vi "Format Fiducial Data.vi"(8 "error in":errorcluster, 9 "Module-Chuck Fiducials":T5(array[cluster]), 10 "Worktable":refnum<class "WorkTable Class.lvclass">, 11 "Console Log in":refnum<class "Console Log.lvclass">) -> (0 "error out":errorcluster, 2 "Formatted Fiducial Data":string, 3 "Console Log out":refnum<class "Console Log.lvclass">)   [LabVIEW 2011, in "Console Log.lvclass"]
uses:
  Console Log.lvclass
  Shared Components/Utils/Type Definitions/Fiducial Image.ctl
  Shared Components/Vec3d Class/Vec3d Class.lvclass
  Shared Components/Utils/Type Definitions/Physical Image.ctl
  <vilib>/vision/Image Controls.llb/IMAQ Image.ctl
  Shared Components/Utils/Type Definitions/Fiducial with Source.ctl
  Shared Components/WorkTable Class/WorkTable Class.lvclass
  Shared Components/Config Manager Class/Type Definitions/Part Type.ctl
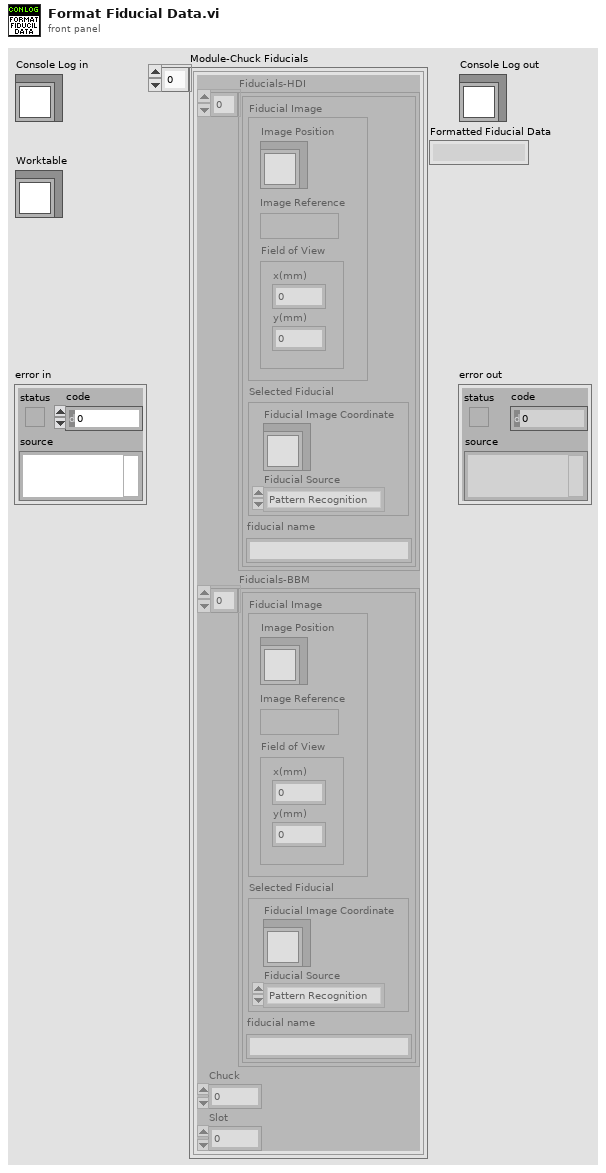
[diagram p1: front panel]
types:
  T1 = typedef "Fiducial Image.ctl" = cluster{"Fiducial Image":T2, "Selected Fiducial":T4, "fiducial name":string}
  T2 = typedef "Physical Image.ctl" = cluster{"Image Position":refnum<class "Vec3d Class.lvclass">, "Image Reference":T3, "Field of View":cluster{"x(mm)":dbl, "y(mm)":dbl}}
  T3 = typedef "IMAQ Image.ctl" = refnum<image>
  T4 = typedef "Fiducial with Source.ctl" = cluster{"Fiducial Image Coordinate":refnum<class "Vec3d Class.lvclass">, "Fiducial Source":enum16{"Pattern Recognition", "User", "Error", "Default"}}
  T5 = cluster{"Fiducials-HDI":T1[], "Fiducials-BBM":T1[], "Chuck":i32, "Slot":i32}[]
  T6 = typedef "Part Type.ctl" = enum16{"BBM", "HDI", "GLUERESERVOIR", "STAMP", "WEIGHT"}
  T7 = typedef "Worktable_Module Slot.ctl" = cluster{"Slot State":enum16{"Empty", "Unglued", "Stamped", "PartOnTop", "Weighted", "Unpotted", "Potted"}, "BBM Type":enum16{"None", "BBM", "GlassSlide"}, "HDI Type":enum16{"None", "HDI", "Polyimide"}, "Vacuum Channel":u8, "Location/Orientation BBM":T8, "Location/Orientation HDI":T8, "S/N":string}
  T8 = typedef "Position_Orientation.ctl" = cluster{"Center":refnum<class "Vec3d Class.lvclass">, "Orientation":refnum<class "Orient3d Class.lvclass">}
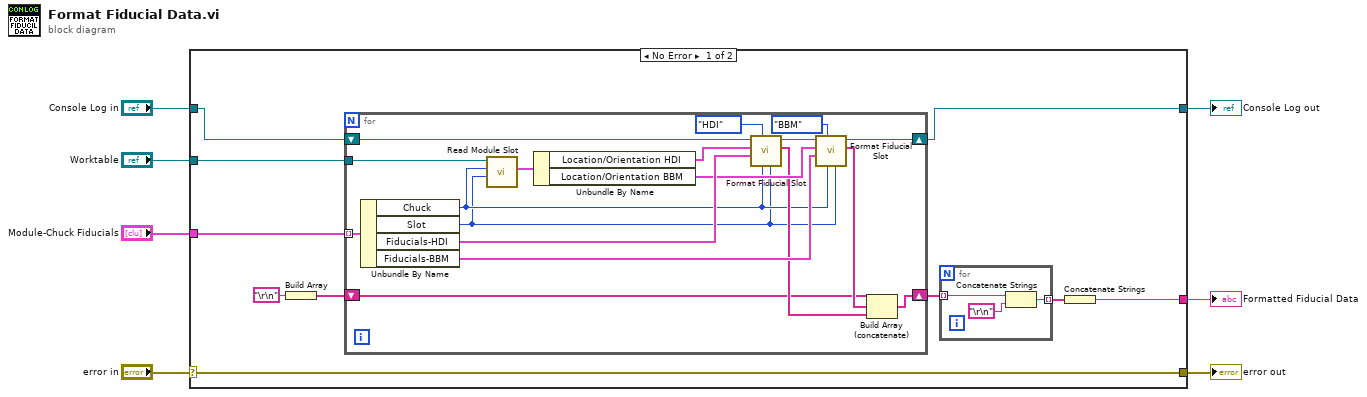
[diagram p0: block diagram]
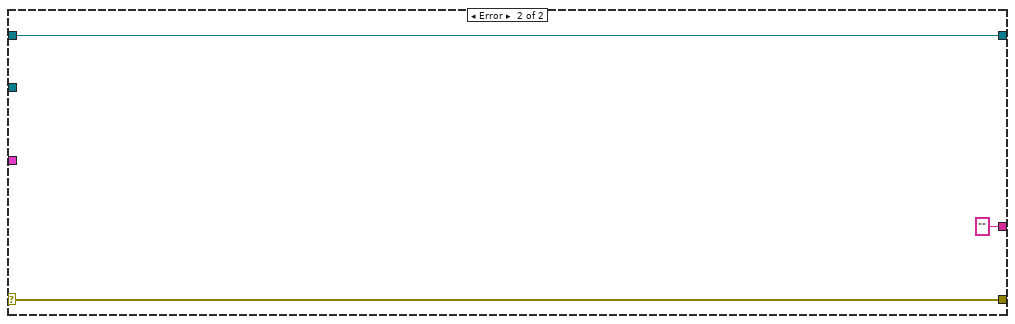
[diagram p2: hidden frame]
diagram:
  n1 = case shown="No Error" "error in" {
    selector: "error in" -> [w17 w41]
    tunnel: [w17 w41] -> w6
    tunnel: [w13 w40] -> w4
    tunnel: "Console Log in" -> [w14 w40]
    tunnel: "Module-Chuck Fiducials" -> [w16 _]
    tunnel: "Worktable" -> [w15 _]
    tunnel: [w10 ""] -> w1
    frame No Error {
      n2 = Build Array("\r\n") -> (w8:string[])
      n3 = for {
        tunnel: w16 -> [w37] mode=indexing
        tunnel: w15 -> [w38]
        shift-right: [w31] -> w13
        shift-left: w14 -> [w33]
        shift-right: [w25] -> w12
        shift-left: w8 -> [w26]
        n4 = Unbundle By Name(w37) -> ("Chuck"=w24:i32, "Slot"=w23:i32, "Fiducials-HDI"=w34:T1[], "Fiducials-BBM"=w29:T1[])
        n5 = call-dynamic "Read Module Slot.vi"("slot"=w23, "chuck"=w24, "WorkTable in"=w38) -> ("Module Slot"=w36:T7)  [unwired: 6 in, 2 out]
        n6 = Unbundle By Name(w36) -> ("Location/Orientation HDI"=w35:T8, "Location/Orientation BBM"=w30:T8)
        n7 = call "Format Fiducial Slot.vi"("Slot"=w23, "Chuck"=w24, "Part Type"=Part_Type."HDI", "Fiducials"=w34, "Location/Orientation"=w35, "Console Log in"=w33) -> ("Array"=w27:string[], "Console Log out"=w32:refnum<class "Console Log.lvclass">)  [unwired: 3 in, 1 out]
        n8 = call "Format Fiducial Slot.vi"("Slot"=w23, "Chuck"=w24, "Part Type"=Part_Type."BBM", "Fiducials"=w29, "Location/Orientation"=w30, "Console Log in"=w32) -> ("Array"=w28:string[], "Console Log out"=w31:refnum<class "Console Log.lvclass">)  [unwired: 3 in, 1 out]
        n9 = Build Array (concatenate)(w26, w28, w27) -> (w25:string[])
      }
      n10 = for {
        tunnel: w12 -> [w20] mode=indexing
        tunnel: [w19] -> w11 mode=indexing
        n11 = Concatenate Strings(w20, "\r\n") -> (w19:string)
      }
      n12 = Concatenate Strings(w11) -> (w10:string)
    }
    frame Error {
    }
  }
  "error out" <- w6
  "Console Log out" <- w4
  "Formatted Fiducial Data" <- w1
